vi "BK Precision 5491B Acquire Continuous Reading.vi"() -> ()   [LabVIEW 2014]
doc: "This example shows how to configure primary and secondary measurement functions and read continuously."
uses:
  <instrlib>/BK Precision 5491B/BK Precision 5491B.lvlib
panel:
  in  "stop":bool
  in  "Secondary Function (1: AC Volts)":u16(ring)=1 items=["DC Volts", "AC Volts", "DC Current", "AC Current", "Frequency", "dB", "dBm"]
  in  "Auto Range (T:Enable)":bool=TRUE
  in  "Manual Range (1000)":dbl=1000.0 format="%#.3f"
  in  "Primary Function (0: DC Volts)":u16(ring) items=["DC Volts", "AC Volts", "AC+DC Volts", "DC Current", "AC Current", "AC+DC Current", "2-Wire Resistance", "Frequency", "Period", "Diode", "Continuity"]
  out "Secondary Measurement":dbl
  out "Primary Measurement":dbl
  in  "Serial Configuration":T1={"Baud Rate"=9600, "Parity"=0, "Data Bits"=8, "Stop Bits"=10, "Flow Control"=0} {"Flow Control" items=["None", "XON/XOFF", "RTS/CTS", "XON/XOFF & RTS/CTS", "DTR/DSR", "XON/XOFF & DTR/DSR"]; "Stop Bits" items=["1.0"=10, "1.5"=15, "2.0"=20]; "Data Bits" items=["8"=8]; "Parity" items=["None", "Odd", "Even", "Mark", "Space"]; "Baud Rate" items=["4800"=4800, "9600"=9600, "19200"=19200, "38400"=38400]}
  in  "VISA resource name":refnum<visa-resource-name>
  # "(c) 2016 B&K Precision Corporation.  ALL RIGHTS RESERVED."
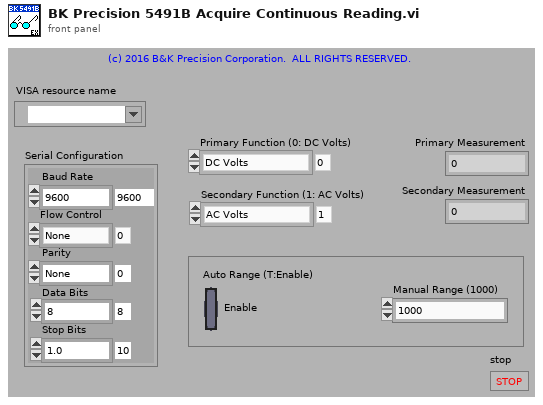
[diagram p1: front panel]
types:
  T1 = cluster{"Baud Rate":u32, "Parity":u16, "Data Bits":u16, "Stop Bits":u16, "Flow Control":u16}
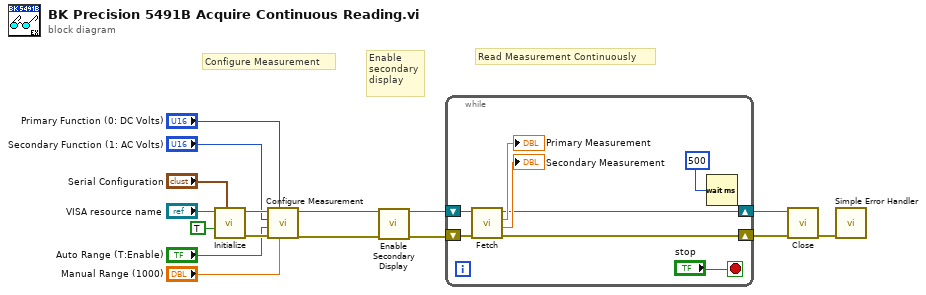
[diagram p0: block diagram]
diagram:
  # "Enable\nsecondary\ndisplay"
  # "Read Measurement Continuously"
  # "Configure Measurement"
  n1 = call <instrlib>:"Initialize.vi"("Serial Configuration"="Serial Configuration", "Reset (True)"=TRUE, "VISA resource name"="VISA resource name") -> ("error out"=w13:errorcluster, "VISA resource name out"=w14:refnum<visa-resource-name>)  [unwired: 7 in]
  n2 = call <instrlib>:"Configure Measurement.vi"("Manual Range (1000)"="Manual Range (1000)", "Primary Function (0: DC Volts)"="Primary Function (0: DC Volts)", "error in (no error)"=w13, "Auto Range (T:Enable)"="Auto Range (T:Enable)", "Secondary Function (1: AC Volts)"="Secondary Function (1: AC Volts)", "VISA resource name"=w14) -> ("error out"=w3:errorcluster, "VISA resource name out"=w4:refnum<visa-resource-name>)  [unwired: 4 in]
  n3 = call <instrlib>:"Enable Secondary Display.vi"("error in (no error)"=w3, "VISA resource name"=w4) -> ("error out"=w2:errorcluster, "VISA resource name out"=w1:refnum<visa-resource-name>)  [unwired: 8 in]
  n4 = while {
    shift-right: [w20] -> w11
    shift-left: w1 -> [w24]
    shift-right: [w19] -> w12
    shift-left: w2 -> [w23]
    stop <- "stop" stop-if-true
    n5 = call <instrlib>:"Fetch.vi"("error in (no error)"=w23, "VISA resource name"=w24) -> ("error out"=w19:errorcluster, "Secondary Measurement"=→"Secondary Measurement":dbl, "Primary Measurement"=→"Primary Measurement":dbl, "VISA resource name out"=w20:refnum<visa-resource-name>)  [unwired: 6 in]
    n6 = Wait (ms)(milliseconds to wait=u32 500 ("Delay Time (0)")) -> ()  [unwired: 1 out]
  }
  n7 = call <instrlib>:"Close.vi"("error in (no error)"=w12, "VISA resource name"=w11) -> ("error out"=w16:errorcluster)  [unwired: 9 in]
  n8 = call <vilib>:"Simple Error Handler.vi"("error in (no error)"=w16) -> ()  [unwired: 4 in, 5 out]
